vi "Read Transpose Array.vi"(9 "GraphChart in":refnum<class "GraphChart.lvclass">) -> (3 "GraphChart out":refnum<class "GraphChart.lvclass">, 4 "Transpose Array":bool)   [LabVIEW 2014, in "GraphChart.lvclass"]
uses:
  GraphChart.lvclass
  GraphChart.lvclass/GraphChart.ctl
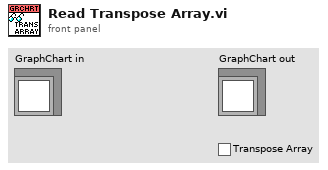
[diagram p1: front panel]
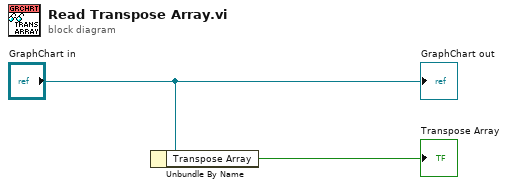
[diagram p0: block diagram]
diagram:
  n1 = Unbundle By Name("GraphChart in") -> ("Transpose Array"=→"Transpose Array":bool)
  "GraphChart out" <- "GraphChart in"
